vi "EF_Initialize.vi"(11 "path":path) -> (0 "EF_DAQThread_IniData":T6, 1 "EF_DAQThread_Data":T7, 2 "EF_AllQRefs":T1, 5 "ExitRef":refnum<event-registration>, 7 "Exit":refnum<user-event>)   [LabVIEW 2017]
uses:
  Types/EF_DAQThread_Data.ctl
  _lib/PQ/PicoHarp/PH_InitInfo.ctl
  Types/EF_GUIThread_IniData.ctl
  Types/EF_AllQRefs.ctl
  Types/EF_GUIThread_QRef.ctl
  Types/EF_GUIThread_QData.ctl
  Types/EF_GUIThread_QCmds.ctl
  Types/EF_DAQThread_QRef.ctl
  Types/EF_DAQThread_QData.ctl
  Types/EF_DAQThread_QCmds.ctl
  Types/EF_DataProcThread_QRef.ctl
  Types/EF_DataProcThread_QData.ctl
  Types/EF_DataProcThread_QCmds.ctl
  Types/EF_AnalysisThread_QRef.ctl
  Types/EF_AnalysisThread_QData.ctl
  Types/EF_AnalysisThread_QCmds.ctl
  _lib/PQ/PicoHarp/phlib_x86_x64_AnyThread.llb/PH_DllPath_global.vi
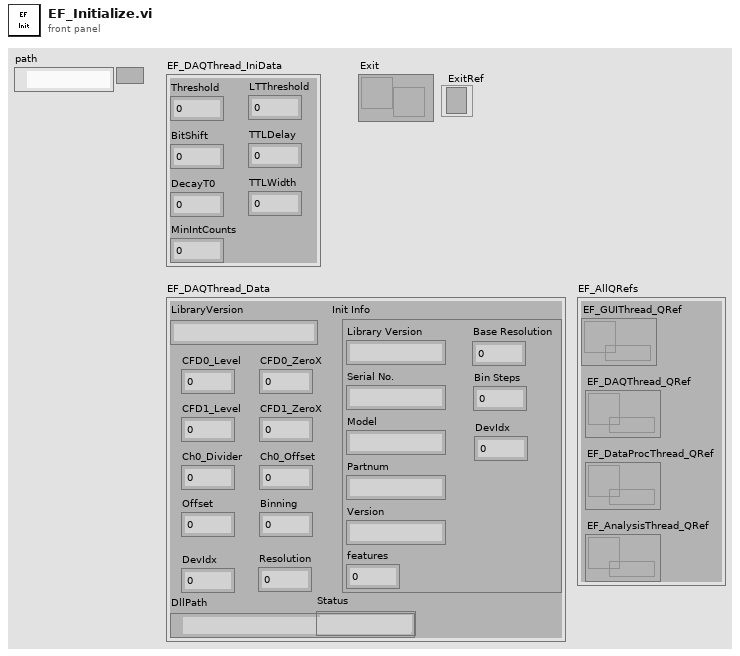
[diagram p1: front panel]
types:
  T1 = typedef "EF_AllQRefs.ctl" = cluster{"EF_GUIThread_QRef":T2, "EF_DAQThread_QRef":T3, "EF_DataProcThread_QRef":T4, "EF_AnalysisThread_QRef":T5}
  T2 = typedef "EF_GUIThread_QRef.ctl" = refnum<queue>
  T3 = typedef "EF_DAQThread_QRef.ctl" = refnum<queue>
  T4 = typedef "EF_DataProcThread_QRef.ctl" = refnum<queue>
  T5 = typedef "EF_AnalysisThread_QRef.ctl" = refnum<queue>
  T6 = typedef "EF_GUIThread_IniData.ctl" = cluster{"Threshold":i32, "BitShift":i32, "DecayT0":dbl, "LTThreshold":dbl, "TTLDelay":i32, "TTLWidth":i32, "MinIntCounts":u32}
  T7 = typedef "EF_DAQThread_Data.ctl" = cluster{"LibraryVersion":string, "CFD0_Level":i32, "CFD0_ZeroX":i32, "CFD1_Level":i32, "CFD1_ZeroX":i32, "Ch0_Divider":i32, "Ch0_Offset":i32, "Init Info":T8, "DevIdx":i32, "Offset":i32, "Binning":i32, "Resolution":dbl, "DllPath":path, "Status":string}
  T8 = typedef "PH_InitInfo.ctl" = cluster{"Library Version":string, "Serial No.":string, "Model":string, "Partnum":string, "Version":string, "features":i32, "Base Resolution":dbl, "Bin Steps":i32, "DevIdx":i32}
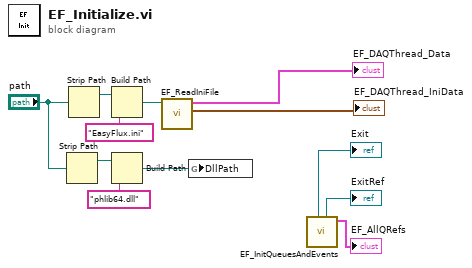
[diagram p0: block diagram]
diagram:
  n1 = Strip Path(path="path") -> (stripped path=w7:path)  [unwired: 1 out]
  n2 = Strip Path(path="path") -> (stripped path=w12:path)  [unwired: 1 out]
  n3 = Build Path(base path=w12, name or relative path="EasyFlux.ini") -> (appended path=w10:path)
  n4 = Build Path(base path=w7, name or relative path="phlib64.dll") -> (appended path=w9:path)
  n5 = call "EF_ReadIniFile.vi"("Path"=w10) -> ("EF_DAQThread_IniData"=→"EF_DAQThread_IniData":T6, "EF_DAQThread_Data"=→"EF_DAQThread_Data":T7)  [unwired: 9 in]
  n6 = global write "PH_DllPath_global.vi" "DllPath"(w9) -> ()
  n7 = call "EF_InitQueuesAndEvents.vi"() -> ("EF_AllQRefs"=→"EF_AllQRefs":T1, "ExitRef"=→"ExitRef":refnum<event-registration>, "Exit"=→"Exit":refnum<user-event>)  [unwired: 9 in]
